vi "Read WiFi MAC.vi"() -> (0 "error out":errorcluster)   [LabVIEW 2020]
panel:
  out "MAC (hexdot string)":string
  in  "Write/Read":i32[](array[ring])=[0] items=["Read", "Write"]
  out "Values Out":dbl[][](array[numeric]) format="%.2f"
  in  "Values In":dbl[][](array[numeric]) format="%.2f"
  in  "NumValues":u16[](array[numeric])=[8]
  in  "Types":u8[](array[numeric])=[99]
  in  "Addresses":u16[](array[numeric])=[60024]
  out "Error String":string
  out "ConnectionType Out":i32
  out "DeviceType Out":i32
  in  "Identifier":string="LJM_idANY"
  in  "ConnectionType":string="LJM_ctANY"
  in  "DeviceType":string="LJM_dtANY"
  out "Error Frame":i32
  # "Older versions of LabVIEW do not\nhave a 64-bit integer, so instead we\nread an array of 8 bytes using\nLJM_eAddresses()."
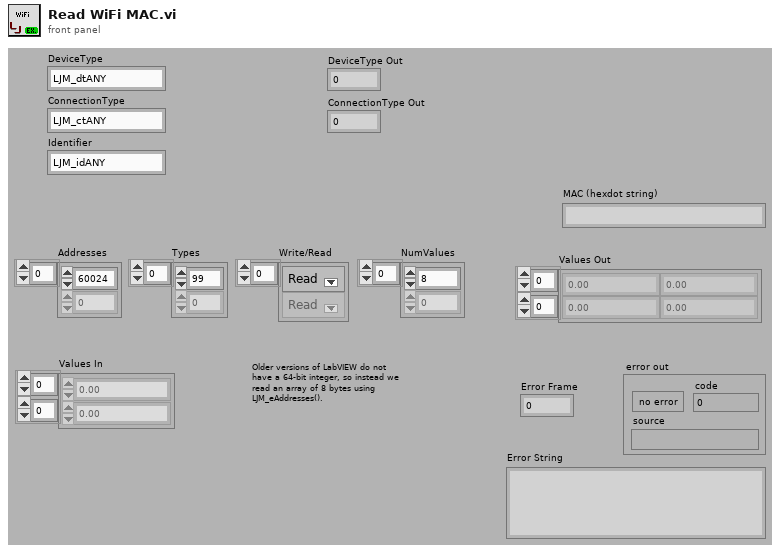
[diagram p1: front panel]
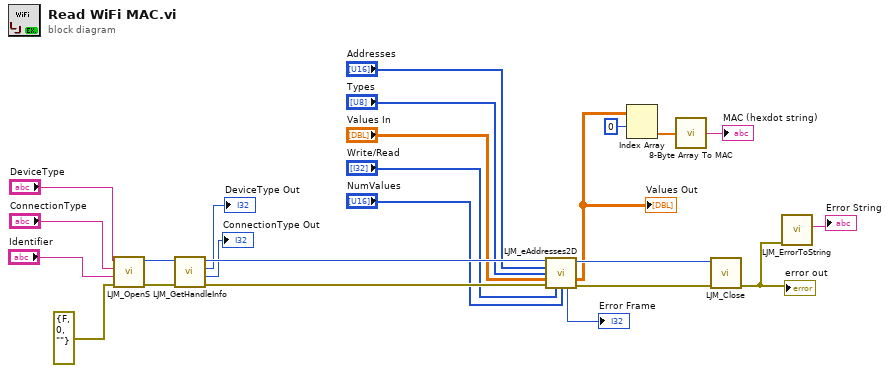
[diagram p0: block diagram]
diagram:
  n1 = call "LJM_OpenS.vi"("error in"=errorcluster {"status"=FALSE, "code"=0, "source"=""} ("error in (no error)"), "Identifier"="Identifier", "ConnectionType"="ConnectionType", "DeviceType"="DeviceType") -> ("error out"=w22:errorcluster, "Handle"=w20:i32)  [unwired: 6 in]
  n2 = call "LJM_GetHandleInfo.vi"("error in"=w22, "Handle In"=w20) -> ("error out"=w21:errorcluster, "ConnectionType"=→"ConnectionType Out":i32, "DeviceType"=→"DeviceType Out":i32, "Handle Out"=w19:i32)  [unwired: 2 in, 4 out]
  n3 = call "LJM_eAddresses2D.vi"("Handle In"=w19, "aAddresses"="Addresses", "aTypes"="Types", "aValuesIn"="Values In", "error in"=w21, "aWrites"="Write/Read", "aNumValues"="NumValues") -> ("Handle Out"=w18:i32, "aValuesOut"=w4:dbl[][], "ErrorAddress"=→"Error Frame":i32, "error out"=w23:errorcluster)  [unwired: 5 in]
  "Values Out" <- w4
  n4 = Index Array(array=w4, index (row)=0) -> (element=w3:dbl[])  [unwired: 1 in]
  n5 = call "8-Byte Array To MAC.vi"("Byte Array"=w3) -> ("MAC (hexdot string)"=→"MAC (hexdot string)":string)
  n6 = call "LJM_Close.vi"("error in"=w23, "Handle"=w18) -> ("error out"=w12:errorcluster)  [unwired: 9 in]
  "error out" <- w12
  n7 = call "LJM_ErrorToString.vi"("error in"=w12) -> ("String"=→"Error String":string)  [unwired: 10 in]
